vi "scoring sensor.vi"(8 "error in":errorcluster) -> ()   [LabVIEW 2023]
uses:
  <vilib>/robotics/Simulator/Engine/ctl/DeviceID.ctl
  <vilib>/Rock Robotics/Network Tables/NT Write Number.vi
  Robot Global Data.vi
  <instrlib>/Devantech SRF05/HAIOL/Devantech SRF05.lvclass
  <vilib>/robotics/Simulator/NI_Robotics_Simulator.lvlib
  <instrlib>/Devantech SRF05/HAIOL/Simulator/Devantech SRF05 Simulator.lvclass
panel:
  out "Waveform Chart":dbl(graph)
  # "This code is added just for simulation scoring.  It increments the score depending on which target a ball passes through. \n\nIt is not expected that you would edit this code.  \n\nWhile this simulation project is not intended to run on a real robot, this code would be removed before building for the roboRIO target."
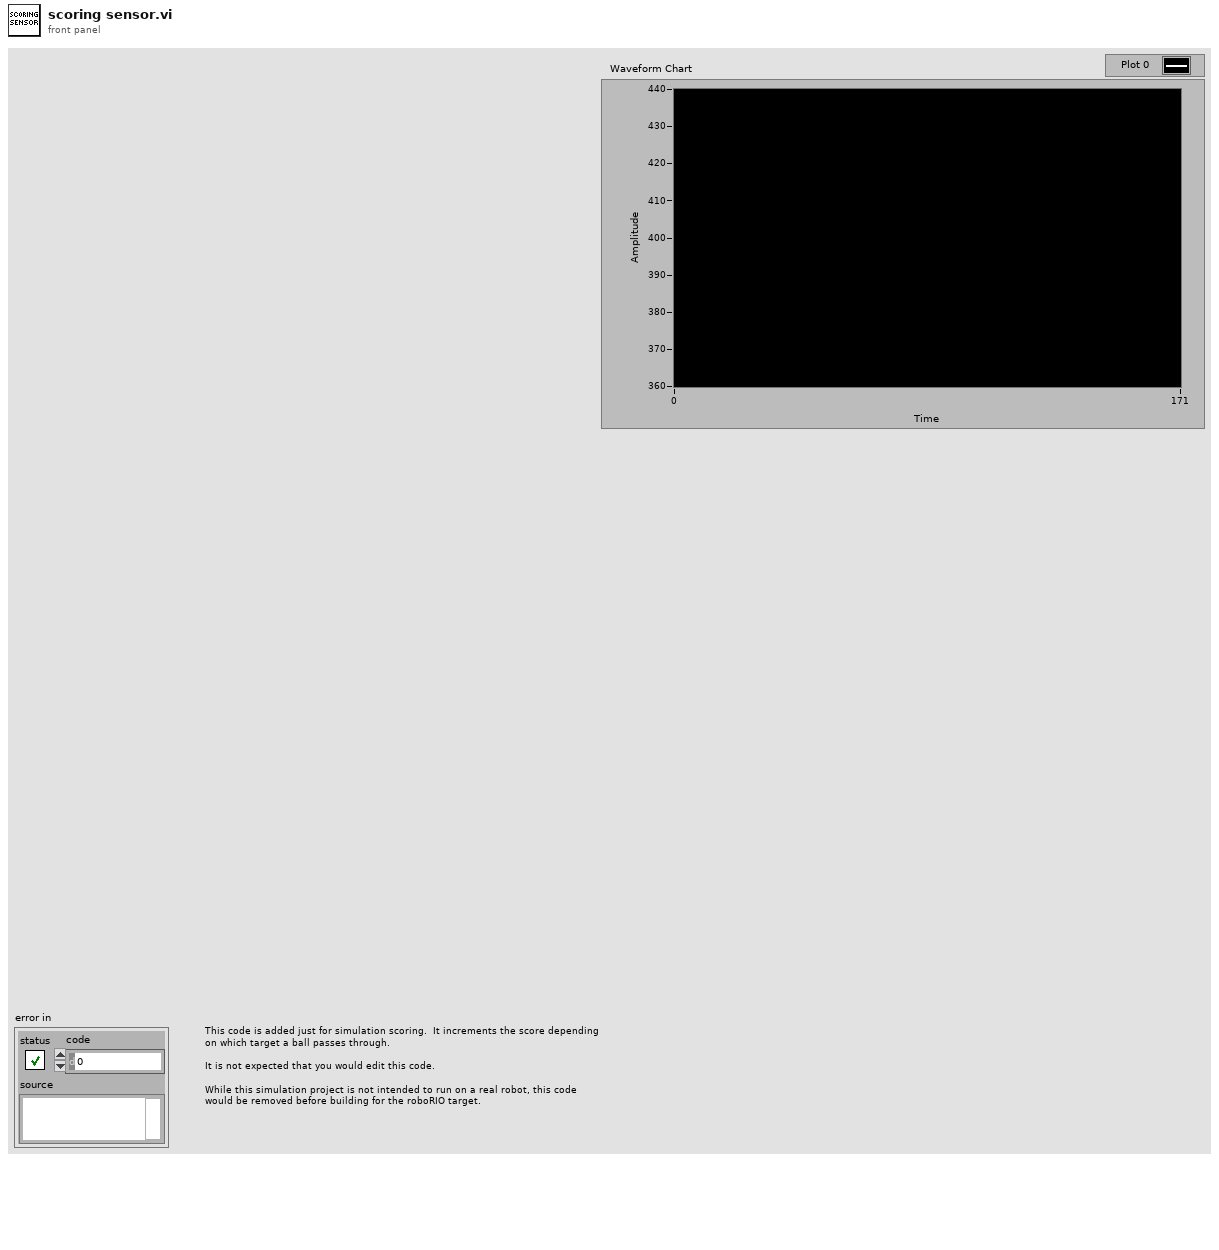
[diagram p1: front panel]
types:
  T1 = typedef "NI_Robotics_Simulator.lvlib/DeviceID.ctl" = cluster{"robot ID":string, "sensor/actuator ID":string}
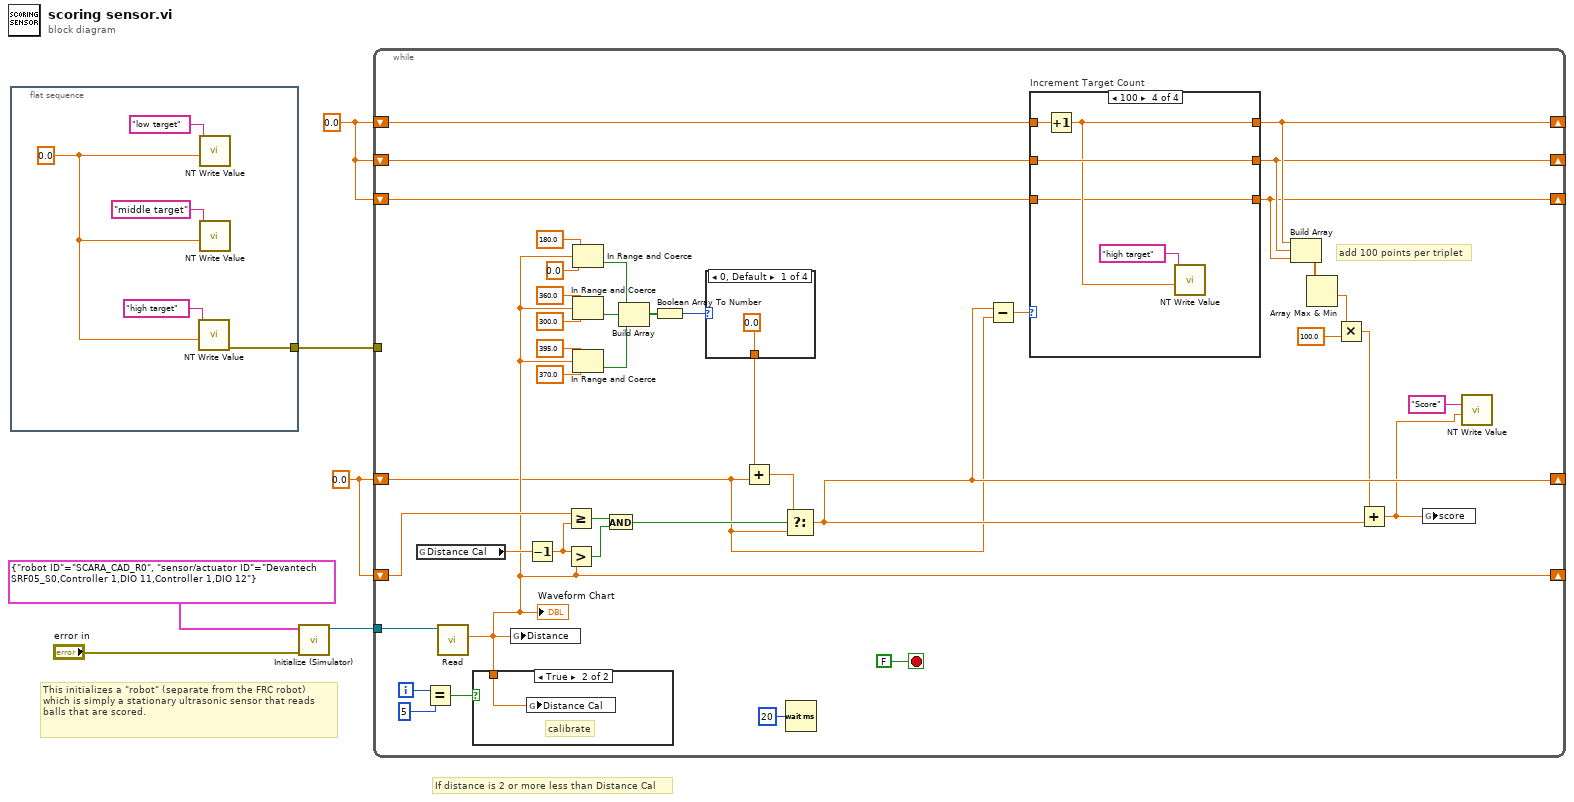
[diagram p0: block diagram]
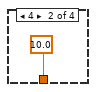
[diagram p2: hidden frame]
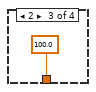
[diagram p3: hidden frame]
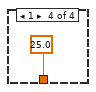
[diagram p4: hidden frame]
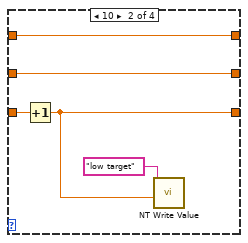
[diagram p6: hidden frame]
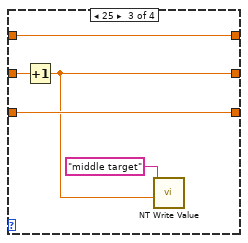
[diagram p7: hidden frame]
diagram:
  w2 = 0.0 ("s? t:f")
  w6 = 0.0 ("score")
  # "This initializes a \"robot\" (separate from the FRC robot) which is simply a stationary ultrasonic sensor that reads balls that are scored."
  # "If distance is 2 or more less than Distance Cal"
  n1 = flat-sequence {
    tunnel: [w8] -> w1
    frame #0 {
      w7 = 0.0 ("Numeric")
      n2 = call-poly <vilib>:"NT Write Value.vi"("value"=w7, "name"="high target" ("Name")) -> ("error out"=w8:errorcluster)  [unwired: 9 in]
      n3 = call-poly <vilib>:"NT Write Value.vi"("value"=w7, "name"="low target" ("Name")) -> ()  [unwired: 9 in, 1 out]
      n4 = call-poly <vilib>:"NT Write Value.vi"("value"=w7, "name"="middle target" ("Name")) -> ()  [unwired: 9 in, 1 out]
    }
  }
  n5 = call <instrlib>:"Initialize (Simulator).vi"("error in (no error)"="error in", "Device ID"=T1 {"robot ID"="SCARA_CAD_R0", "sensor/actuator ID"="Devantech SRF05_S0,Controller 1,DIO 11,Controller 1,DIO 12"}) -> ("Devantech SRF05 out"=w4:refnum<class "Devantech SRF05.lvclass">)  [unwired: 8 in, 1 out]
  n6 = while {
    tunnel: w4 -> [w52]
    shift-right: [w33] -> _
    shift-left: w6 -> [w44]
    shift-right: [w21] -> _
    shift-left: w6 -> [w20]
    shift-right: [w19] -> _
    shift-left: w2 -> [w27]
    shift-right: [w18] -> _
    shift-left: w2 -> [w26]
    shift-right: [w17] -> _
    shift-left: w2 -> [w25]
    tunnel: w1 -> [_]
    i -> [w49]
    stop <- FALSE stop-if-true
    # "add 100 points per triplet"
    n7 = global read "Robot Global Data.vi" "Distance Cal"() -> (w46:dbl)
    n8 = Equal?(x=w49, y=5) -> (x = y?=w47:bool)
    n9 = call-dynamic "Read.vi"("Devantech SRF05 in"=w52) -> ("Distance (cm)"=w33:dbl)  [unwired: 7 in, 3 out]
    "Waveform Chart" <- w33
    n10 = case shown="True" w47 {
      tunnel: w33 -> [_ w75]
      frame False {
      }
      frame True {
        # "calibrate"
        n11 = global write "Robot Global Data.vi" "Distance Cal"(w75) -> ()
      }
    }
    n12 = global write "Robot Global Data.vi" "Distance"(w33) -> ()
    n13 = Decrement(x=w46) -> (x-1=w43:dbl)
    n14 = Greater Or Equal?(x=w44, y=w43) -> (x >= y?=w42:bool)
    n15 = Greater?(x=w43, y=w33) -> (0:w45:bool)
    n16 = In Range and Coerce(upper limit=180.0, x=w33, lower limit=0.0) -> (In Range?=w31:bool)  [unwired: 1 out]
    n17 = In Range and Coerce(upper limit=360.0, x=w33, lower limit=300.0 ("upper limit")) -> (In Range?=w30:bool)  [unwired: 1 out]
    n18 = In Range and Coerce(upper limit=395.0, x=w33, lower limit=370.0 ("upper limit")) -> (In Range?=w29:bool)  [unwired: 1 out]
    n19 = And(x=w42, y=w45) -> (x .and. y?=w41:bool)
    n20 = Build Array(w31, w30, w29) -> (w32:bool[])
    n21 = Boolean Array To Number(Boolean array=w32) -> (number=w24:u32)
    n22 = case shown="0, Default" w24 {
      tunnel: [0.0 ("x") 10.0 ("x") 100.0 ("x") 25.0 ("x")] -> w23
      frame 0, Default {
      }
      frame 4 {
      }
      frame 2 {
      }
      frame 1 {
      }
    }
    n23 = Add(x=w23, y=w20) -> (x+y=w40:dbl)
    n24 = Select(t=w40, s=w41, f=w20) -> (s? t:f=w21:dbl)
    n25 = Wait (ms)(milliseconds to wait=u32 20) -> ()  [unwired: 1 out]
    n26 = Subtract(x=w21, y=w20) -> (x-y=w22:dbl)
    n27 = case "Increment Target Count" shown="100" w22 {
      tunnel: w27 -> [w59 w62 w67 w72]
      tunnel: [w59 w62 w67 w71] -> w19
      tunnel: w26 -> [w58 w63 w68 w73]
      tunnel: w25 -> [w57 w61 w66 w70]
      tunnel: [w58 w63 w65 w73] -> w18
      tunnel: [w57 w60 w66 w70] -> w17
      frame 0, Default {
      }
      frame 10 {
        n28 = Increment(x=w61) -> (x+1=w60:dbl)
        n29 = call-poly <vilib>:"NT Write Value.vi"("value"=w60, "name"="low target" ("Name")) -> ()  [unwired: 9 in, 1 out]
      }
      frame 25 {
        n30 = Increment(x=w68) -> (x+1=w65:dbl)
        n31 = call-poly <vilib>:"NT Write Value.vi"("value"=w65, "name"="middle target" ("Name")) -> ()  [unwired: 9 in, 1 out]
      }
      frame 100 {
        n32 = Increment(x=w72) -> (x+1=w71:dbl)
        n33 = call-poly <vilib>:"NT Write Value.vi"("value"=w71, "name"="high target" ("Name")) -> ()  [unwired: 9 in, 1 out]
      }
    }
    n34 = Build Array(w19, w18, w17) -> (w16:dbl[])
    n35 = Array Max & Min(array=w16) -> (min value=w15:dbl)  [unwired: 3 out]
    n36 = Multiply(x=w15, y=100.0) -> (x*y=w13:dbl)
    n37 = Add(x=w13, y=w21) -> (x+y=w12:dbl)
    n38 = global write "Robot Global Data.vi" "score"(w12) -> ()
    n39 = call-poly <vilib>:"NT Write Value.vi"("value"=w12, "name"="Score" ("Name")) -> ()  [unwired: 9 in, 1 out]
  }
